vi "SRV_Number of Motor Control Buttons.vi"() -> (8 "Number of Motor Control Buttons":i32, 10 "Number of Columns":i32=7)   [LabVIEW 2009]
doc: "Contains the version of the software to display on GUIs.\n\n\nAuthor: Mike Schultz - Logic PD"
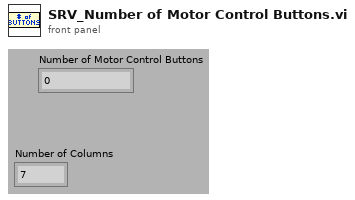
[diagram p1: front panel]
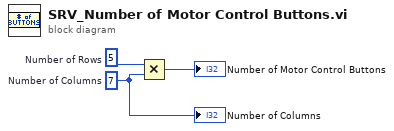
[diagram p0: block diagram]
diagram:
  w2 = 7  # Number of Columns
  w3 = 5  # Number of Rows
  n1 = Multiply(x=w3, y=w2) -> (x*y=→"Number of Motor Control Buttons":i32)
  "Number of Columns" <- w2
